vi "CRYMessage Name Insert.vi"(7 "Setup in":T1={"No.VI"=0, "Category"="", "StepName"="", "Seq setup flattened"="", "Comment"="", "Steps config."=[], "Jump config"=[], "Start"=0.0, "Increment"=0.0, "Name"="Pa", "Unit"="Pa", "Y data"=1, "Y prefix"="", "Y dB ref"=1.0, "Y unit"="", "Repeat State Array"=[]} {"Repeat State Array"."Start" format="%#_5g"; "Y dB ref" format="%.1f"; "Y data" items=["dB", "Lin"]; "Start" format="%#_5g"}, 8 "Hardware setup  in":string, 9 "Step setup in":string, 11 "Type In":string) -> ()   [LabVIEW 2013]
uses:
  Typedef Control/CRYStep.ctl
  Typedef Control/CRYData Cluster.ctl
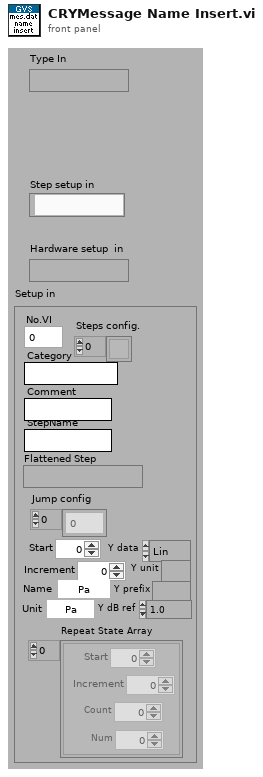
[diagram p1: front panel]
types:
  T1 = typedef "CRYStep.ctl" = cluster{"No.VI":i32, "Category":string, "StepName":string, "Seq setup flattened":string, "Comment":string, "Steps config.":bool[], "Jump config":i32[], "Start":dbl, "Increment":dbl, "Name":string, "Unit":string, "Y data":u16, "Y prefix":string, "Y dB ref":dbl, "Y unit":string, "Repeat State Array":cluster{"Start":dbl, "Increment":dbl, "Count":i32, "Num":i32}[]}
  T2 = cluster{"Start":dbl, "Increment":dbl, "Count":i32, "Num":i32}[]
  T3 = typedef "CRYMessages Cluster.ctl" = cluster{"Name":string, "Type":u16, "Command Msg":string, "Flags":u16, "Dialog?":bool, "Numeric?":bool, "Wait?":bool, "Pause [ms]":i32, "pattern":u32, "Address":string, "Operation":i32, "bytes":i32, "Line selected":u32, "RS232 Func":u16, "Serial Ctrl lines":u16, "Interf #":u8, "GPIB func":u16, "GPIB cmd":u16, "GPIB rem en":bool, "GPIB term":i32, "Curves generated":string[], "Units":cluster{"unit":string, "dB ref":dbl, "axis":u16, "data":u16, "Common dB ref.":u16}, "Axis":u16, "Default Value":dbl, "Message Tilte":string, "Port #":i32, "Print Unit":string, "Text Format":cluster{"Size":u32, "Plain":bool, "Bold":bool, "Italic":bool, "Underline":bool, "Strikethrough":bool, "Color":u32, "Font":string}, "Help":string, "Tab Value":enum32{"Setting", "Help"}, "pattern 2":u32, "Line selected 2":u32, "H_Bits":cluster{"Bits":string[], "Invert":bool, "All":bool}[], "G_Bits":cluster{"Bits":string[], "Invert":bool, "All":bool}[]}
  T4 = typedef "CRYData Cluster.ctl" = cluster{"Name":string, "Curve":cluster{"x":dbl, "y":dbl, "z":dbl}[], "X data":u16, "Y data":u16, "Z data":u16, "X axis":u16, "Y axis":u16, "Z axis":u16, "X unit":string, "Y unit":string, "Z unit":string, "X dB ref":dbl, "Y dB ref":dbl, "Z dB ref":dbl, "single val":bool, "protected":bool, "display X":bool, "display Y":bool, "display Z":bool, "Test Info":string, "Step No.":i32, "Plot Settings":cluster{"Color":u32, "Interpolation":u8, "Point Style":u8, "Line Style":u8, "Point Color":u32, "Line Width":u8, "Bar Plot Style":u8, "Fill To":i16}, "AutoProtect":bool}
  T5 = cluster{"unit":string, "dB ref":dbl, "axis":u16, "data":u16, "Common dB ref.":u16}
  T6 = cluster{"Default Value":dbl, "Numeric Entry":dbl, "Numeric Entry":dbl}
  T7 = cluster{"Numeric":dbl, "Default Value":dbl, "Numeric":dbl}
  T8 = cluster{"Numeric Entry":dbl, "Numeric Entry":dbl, "Default Value":dbl}
  T9 = cluster{"Numeric Entry":dbl, "Numeric Entry":dbl, "Default Value":dbl}[]
  T10 = typedef "CRYResult Cluster.ctl" = cluster{"Name":string, "Margin":dbl, "unit":string, "Verdict":bool, "Limit":string, "Max/Min":string, "protected":bool, "Step No.":i32, "Test Info":string, "AutoProtect":bool}
  T11 = typedef "CRYData Cluster Array.ctl" = T4[]
  T12 = typedef "CRYResult Cluster Array.ctl" = T10[]
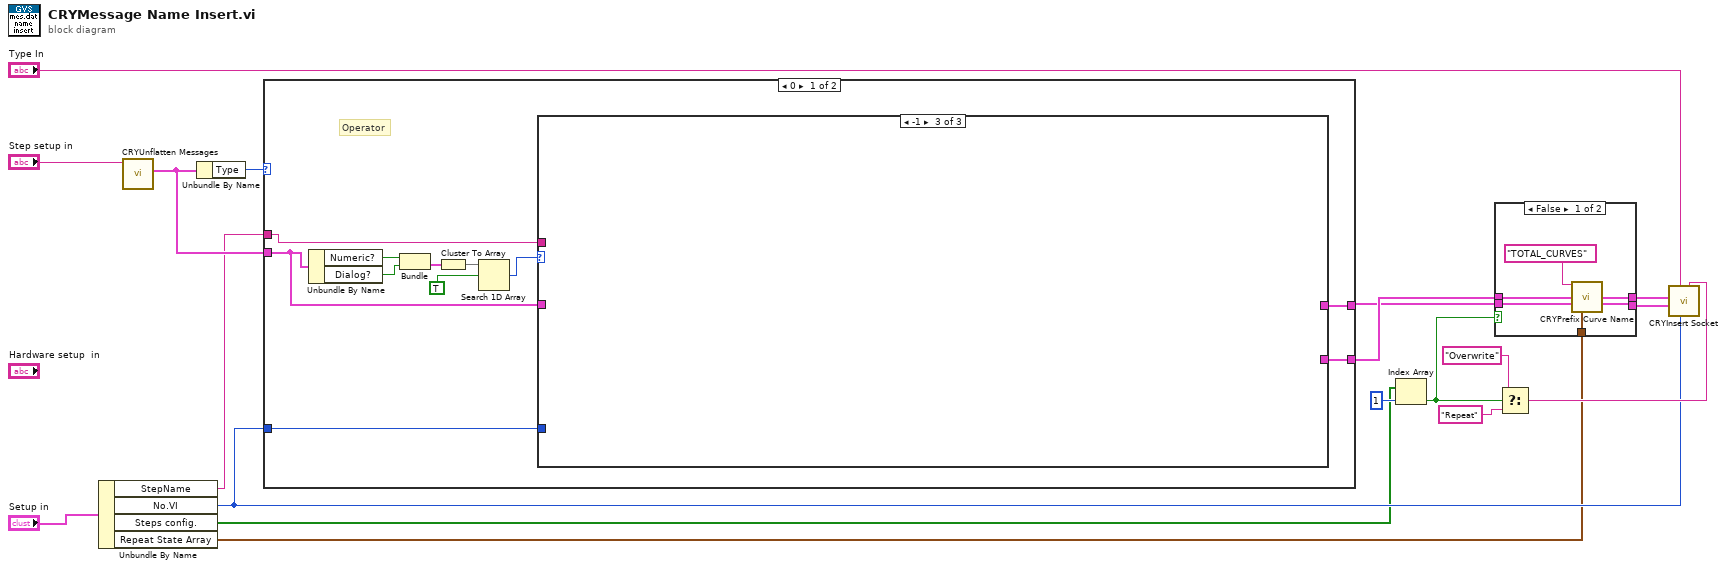
[diagram p0: block diagram]
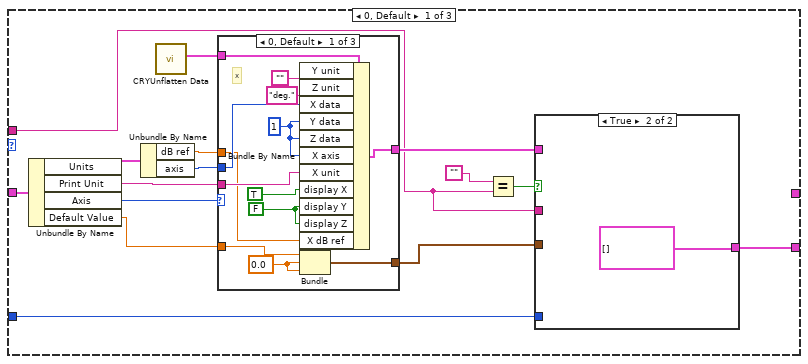
[diagram p3: hidden frame]
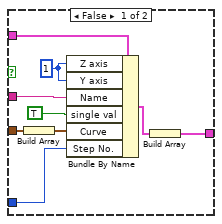
[diagram p4: hidden frame]
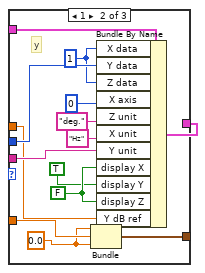
[diagram p5: hidden frame]
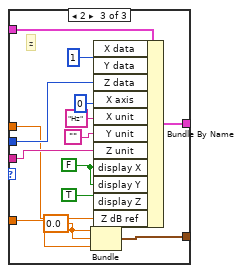
[diagram p6: hidden frame]
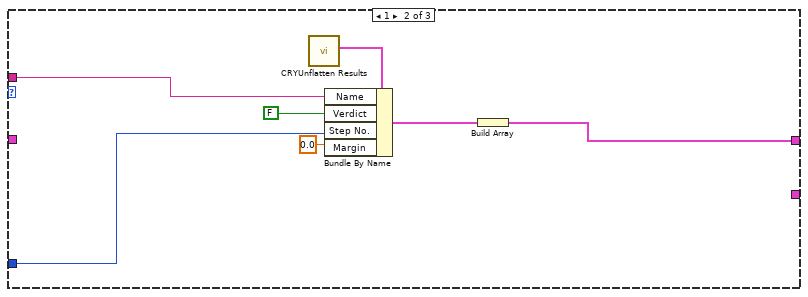
[diagram p7: hidden frame]
diagram:
  n1 = Unbundle By Name("Setup in") -> ("StepName"=w1:string, "No.VI"=w9:i32, "Steps config."=w8:bool[], "Repeat State Array"=w2:T2)
  n2 = call "CRYUnflatten Messages.vi"("Unflatten Messages"="Step setup in") -> ("Messages"=w17:T3)  [unwired: 10 out]
  n3 = Unbundle By Name(w17) -> ("Type"=w16:u16)
  n4 = case shown="0" w16 {
    tunnel: w17 -> [w21 _]
    tunnel: w9 -> [w29 _]
    tunnel: [w28 _] -> w7
    tunnel: [w20 _] -> w6
    tunnel: w1 -> [w19 _]
    frame 0 {
      # "Operator"
      n5 = Unbundle By Name(w21) -> ("Numeric?"=w24:bool, "Dialog?"=w23:bool)
      n6 = Bundle("Numeric?"=w24, "Dialog?"=w23) -> (w26:cluster{"Numeric?":bool, "Dialog?":bool})  [unwired: 1 out]
      n7 = Cluster To Array(cluster=w26) -> (array=w25:bool[])
      n8 = Search 1D Array(1D array=w25, element=TRUE) -> (index of element=w22:i32)  [unwired: 1 out]
      n9 = case shown="-1" w22 {
        tunnel: w21 -> [w44 _ _]
        tunnel: w29 -> [w35 w96 _]
        tunnel: [w33 _ _] -> w28
        tunnel: w19 -> [w30 w99 _]
        tunnel: [_ w98 _] -> w20
        frame 0, Default {
          n10 = Unbundle By Name(w44) -> ("Units"=w39:T5, "Print Unit"=w38:string, "Axis"=w37:u16, "Default Value"=w34:dbl)
          n11 = Unbundle By Name(w39) -> ("dB ref"=w36:dbl, "axis"=w40:u16)
          n12 = call "CRYUnflatten Data.vi"() -> ("Datum"=w42:T4)  [unwired: 1 in, 10 out]
          n13 = case shown="0, Default" w37 {
            tunnel: [w67 w81 w95] -> w41
            tunnel: w34 -> [w65 w77 w90]
            tunnel: w42 -> [w64 w80 w94]
            tunnel: [w63 w79 w93] -> w43
            tunnel: w38 -> [w62 w78 w92]
            tunnel: w40 -> [w56 w72 w84]
            tunnel: w36 -> [w55 w68 w82]
            frame 0, Default {
              w59 = u16 1 ("Y data")
              w60 = FALSE ("display Y")
              w66 = 0.0 ("Numeric Entry")
              # "x"
              n14 = Bundle By Name(cluster=w64, "Y unit"="", "Z unit"="deg.", "X data"=w56, "Y data"=w59, "Z data"=w59, "X axis"=w59, "X unit"=w62, "display X"=TRUE, "display Y"=w60, "display Z"=w60, "X dB ref"=w55) -> (w63:T4)
              n15 = Bundle("Default Value"=w65, "Numeric Entry"=w66, "Numeric Entry"=w66) -> (w67:T6)  [unwired: 1 out]
            }
            frame 1 {
              w69 = 0.0 ("Numeric")
              w71 = u16 1 ("X data")
              w76 = FALSE ("display X")
              # "y"
              n16 = Bundle("Numeric"=w69, "Default Value"=w77, "Numeric"=w69) -> (w81:T7)  [unwired: 1 out]
              n17 = Bundle By Name(cluster=w80, "X data"=w71, "Y data"=w72, "Z data"=w71, "X axis"=u16 0, "Z unit"="deg.", "X unit"="Hz", "Y unit"=w78, "display X"=w76, "display Y"=TRUE, "display Z"=w76, "Y dB ref"=w68) -> (w79:T4)
            }
            frame 2 {
              w83 = u16 1 ("X data")
              w89 = FALSE ("display X")
              w91 = 0.0 ("Numeric Entry")
              # "z"
              n18 = Bundle("Numeric Entry"=w91, "Numeric Entry"=w91, "Default Value"=w90) -> (w95:T8)  [unwired: 1 out]
              n19 = Bundle By Name(cluster=w94, "X data"=w83, "Y data"=w83, "Z data"=w84, "X axis"=u16 0, "X unit"="Hz", "Y unit"="", "Z unit"=w92, "display X"=w89, "display Y"=w89, "display Z"=TRUE, "Z dB ref"=w82) -> (w93:T4)
            }
          }
          n20 = Equal?(x="", y=w30) -> (x = y?=w31:bool)
          n21 = case shown="True" w31 {
            tunnel: w43 -> [w53 _]
            tunnel: w41 -> [w52 _]
            tunnel: w35 -> [w48 _]
            tunnel: [w47 T4[] []] -> w33
            tunnel: w30 -> [w45 _]
            frame False {
              w49 = u16 1 ("Z axis")
              n22 = Build Array(w52) -> (w50:T9)
              n23 = Bundle By Name(cluster=w53, "Z axis"=w49, "Y axis"=w49, "Name"=w45, "single val"=TRUE ("Bundle Element"), "Curve"=w50, "Step No."=w48) -> (w46:T4)
              n24 = Build Array(w46) -> (w47:T4[])
            }
            frame True {
            }
          }
        }
        frame 1 {
          n25 = call "CRYUnflatten Results.vi"() -> ("Result"=w101:T10)  [unwired: 9 in, 2 out]
          n26 = Bundle By Name(cluster=w101, "Name"=w99, "Verdict"=FALSE, "Step No."=w96, "Margin"=0.0) -> (w97:T10)
          n27 = Build Array(w97) -> (w98:T10[])
        }
        frame -1 {
        }
      }
    }
    frame Default {
    }
  }
  n28 = Index Array(array=w8, index=1) -> (element=w3:bool)
  n29 = case shown="False" w3 {
    tunnel: w7 -> [w107 w110]
    tunnel: w6 -> [w106 w109]
    tunnel: [w105 w110] -> w5
    tunnel: [w104 w109] -> w4
    tunnel: w2 -> [w103 _]
    frame False {
      n30 = call "CRYPrefix Curve Name.vi"("Type In"="TOTAL_CURVES", "Values In"=w107, "Results In"=w106, "Repeat State Array In"=w103) -> ("Values Out"=w105:T11, "Results Out"=w104:T12)  [unwired: 8 in, 2 out]
    }
    frame True {
    }
  }
  n31 = Select(t="Overwrite" ("Y unit"), s=w3, f="Repeat") -> (s? t:f=w11:string)
  n32 = call "CRYInsert Socket.vi"("sOption2"=w11, "Step No."=w9, "sOption1"="Type In", "Results"=w4, "Values"=w5) -> ()  [unwired: 6 in, 1 out]
